vi "Giros_Verticales.vi"   [LabVIEW 2016]
uses:
  <vilib>/imath/engines/lvmath2/RunTimeEngine/RangeToken/NIMS_Range_R3 - Integer.vi
  <instcachedir>/0/NIMS_Range_R3 - Integer_A435E2FF893B4C718FD5055FE39FE2F6.lvgen/NIMS_Range_R3 - Integer_A435E2FF893B4C718FD5055FE39FE2F6_000.vi
  <vilib>/imath/engines/lvmath2/RunTimeEngine/CommandStatement/MC_CommandStatement_break.vi
  <vilib>/imath/engines/lvmath2/RunTimeEngine/ArithmeticOperatorToken/NIMS_ArithmeticOperator_multmx(M,CV)-internal.vi
  <instcachedir>/0/NIMS_ArithmeticOperator_multmx(M,CV)-internal_14A0C3390E0F41A88768D45F6518085A.lvgen/NIMS_ArithmeticOperator_multmx(M,CV)-internal_14A0C3390E0F41A88768D45F6518085A_002.vi
  <vilib>/imathl/engines/lvmath/Functions/Error Handling/Create Error.vi
  <vilib>/imath/engines/lvmath2/RunTimeEngine/VariableToken/NIMS_VariableToken_CondDefinedDefinedByReplace.vi
  <instcachedir>/0/NIMS_VariableToken_CondDefinedDefinedByReplace_D162CFFC24174562A9FEA619A91E1A56.lvgen/NIMS_VariableToken_CondDefinedDefinedByReplace_D162CFFC24174562A9FEA619A91E1A56_001.vi
  <vilib>/imath/engines/lvmath2/RunTimeEngine/IndexRead/NIMS V(S).vi
  <instcachedir>/0/NIMS V(S)_0488751826AF41519A22953C041130DC.lvgen/NIMS V(S)_0488751826AF41519A22953C041130DC_000.vi
  <vilib>/imath/engines/lvmath2/RunTimeEngine/BuiltInFunctions/round/NIMS_round(DBL-S).vi
  <vilib>/imath/engines/lvmath2/RunTimeEngine/IndexReplace/NIMS M(S,S)=S.vi
  <instcachedir>/0/NIMS M(S,S)=S_98E40400474E4398B113AE20298B4F82.lvgen/NIMS M(S,S)=S_98E40400474E4398B113AE20298B4F82_000.vi
  <vilib>/imath/engines/lvmath2/RunTimeEngine/ErrorHandling/NIMS_Create Error From Enums.vi
  <vilib>/imath/engines/lvmath2/RunTimeEngine/VariableToken/NIMS_VariableToken_CondDefined.vi
  <instcachedir>/0/NIMS_VariableToken_CondDefined_06E9DA95BD4D46A6BA55EC651A891960.lvgen/NIMS_VariableToken_CondDefined_06E9DA95BD4D46A6BA55EC651A891960_001.vi
  <vilib>/imath/engines/lvmath/Functions/Error Handling/MergeErrorsWrapper.vi
  <vilib>/imath/engines/lvmath2/RunTimeEngine/NodeEndStatement/NIMS_NodeEndStatement_Output.vi
  <instcachedir>/0/NIMS_NodeEndStatement_Output_53EC0D466D134D7ABD903AC30B43404B.lvgen/NIMS_NodeEndStatement_Output_53EC0D466D134D7ABD903AC30B43404B_012.vi
  <vilib>/imath/engines/lvmath2/RunTimeEngine/ErrorHandling/NIMS_Finalize Error.vi
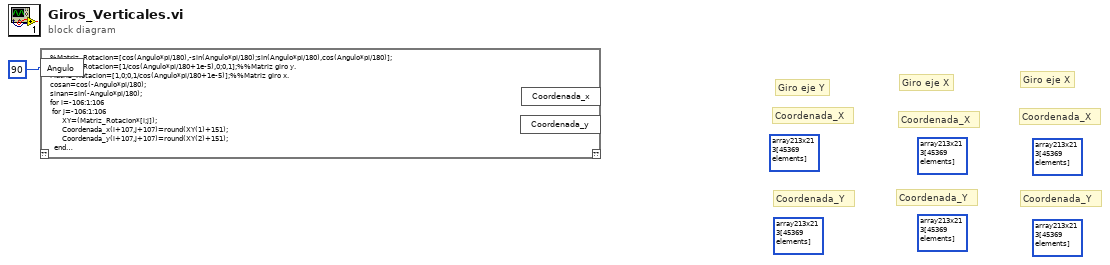
[diagram p0: block diagram]
diagram:
  (unwired) i16[][] array213x213[45369 elements] ("Coordenada_y")
  (unwired) i16[][] array213x213[45369 elements] ("Coordenada_x")
  (unwired) i16[][] array213x213[45369 elements] ("Coordenada_y")
  (unwired) i16[][] array213x213[45369 elements] ("Coordenada_x")
  (unwired) i16[][] array213x213[45369 elements] ("Coordenada_y")
  (unwired) i16[][] array213x213[45369 elements] ("Coordenada_x")
  # "Coordenada_Y"
  # "Giro eje X"
  # "Coordenada_X"
  # "Giro eje X"
  # "Coordenada_X"
  # "Coordenada_Y"
  # "Giro eje Y"
  # "Coordenada_Y"
  # "Coordenada_X"
  n1 = mathscript code="%Matriz_Rotacion=[cos(Angulo*pi/180),-sin(Angulo*pi/180);sin(Angulo*pi/180),cos(Angulo*pi/180)];\n%Matriz_Rotacion=[1/cos(Angulo*pi/180+1e-5),0;0,1];%%Matriz giro y.\nMatriz_Rotacion=[1,0;0,1/cos(Angulo*pi/180+1e-5)];%%Matriz giro x.\ncosan=cos(-Angulo*pi/180);\nsinan=sin(-Angulo*pi/180);\nfor i=-106:1:106\n for j=-106:1:106\n      XY=(Matriz_Rotacion*[i;j]);\n      Coordenada_x(i+107,j+107)=round(XY(1)+151);\n      Coordenada_y(i+107,j+107)=round(XY(2)+151);\n  end\nend\n%for j=1:1:213\n %for i=1:1:213\n %      Coordenada_x(i,j)=round((i-107)*cosan-(j-107)*sinan+151);\n %      Coordenada_y(i,j)=round((i-107)*sinan+(j-107)*cosan+151);\n %end\n%end"("Angulo"=90) -> ()  [unwired: 1 in, 3 out]
